vi "ConfigureWfrm.vi"(8 "error in (no error)":errorcluster, 10 "SampleRate":dbl=1000.0, 11 "PmuTestFunctions in":refnum<class "PmuTestFunctions.lvclass">) -> (0 "error out":errorcluster, 3 "PmuTestFunctions out":refnum<class "PmuTestFunctions.lvclass">)   [LabVIEW 2014, in "Functions.lvlib" / "PmuTestFunctions.lvclass"]
uses:
  PmuTestFunctions.lvclass
  ArbitraryFunction/ArbitraryFunction.lvclass/ArbitraryFunction.ctl
  PmuTestFunctions.lvclass/PmuTestFunctions.ctl
  ArbitraryFunction/Accessors/Read SampleRate.vi
  Accessors/Read PmuTestParams.vi
  Accessors/Read T0.vi
  ArbitraryFunction/Accessors/Read Arbs.vi
  Accessors/Read SettlingTime.vi
  ArbitraryFunction/Accessors/Write Arbs.vi
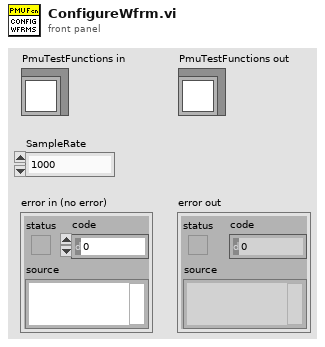
[diagram p1: front panel]
types:
  T1 = typedef "Functions.lvlib/PmuTestFunctions.lvclass/PmuTestParams.ctl" = dbl[][]
  T2 = typedef "Functions.lvlib/ArbitraryFunction.lvclass/Arbitrary.ctl" = cluster{"Handle":string, "Size":i32, "Gain":dbl, "Offset":dbl, "Waveform":waveform(dbl)}
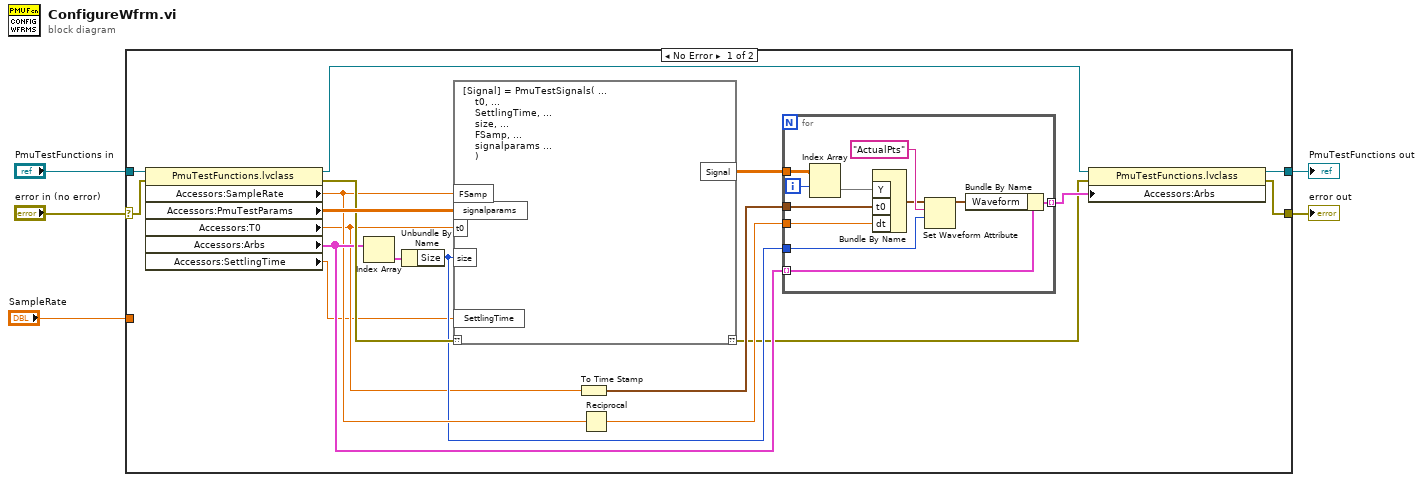
[diagram p0: block diagram]
diagram:
  n1 = case shown="No Error" "error in (no error)" {
    selector: "error in (no error)" -> [w22 w36]
    tunnel: [w7 w36] -> w4
    tunnel: [w8 w35] -> w2
    tunnel: "PmuTestFunctions in" -> [w23 w35]
    tunnel: "SampleRate" -> [_ _]
    frame No Error {
      n2 = property class="PmuTestFunctions.lvclass"(reference=w23, error in=w22) -> (reference out=w11:refnum<class "PmuTestFunctions.lvclass">, error out=w19:errorcluster, "Accessors:SampleRate"=w16:dbl, "Accessors:PmuTestParams"=w20:T1, "Accessors:T0"=w13:dbl, "Accessors:Arbs"=w18:T2[], "Accessors:SettlingTime"=w6:dbl)
      n3 = Index Array(array=w18) -> (element=w21:T2)  [unwired: 1 in]
      n4 = Unbundle By Name(w21) -> ("Size"=w14:i32)
      n5 = script code="[Signal] = PmuTestSignals( ...\n    t0, ...\n    SettlingTime, ...\n    size, ...\n    FSamp, ...\n    signalparams ...\n    )"("??"=w19, "t0"=w13, "size"=w14, "SettlingTime"=w6, "signalparams"=w20, "FSamp"=w16) -> ("??"=w9:errorcluster, "Signal"=w17:dbl[][])
      n6 = To Time Stamp(1:w13) -> (0:w12:timestamp)
      n7 = Reciprocal(x=w16) -> (1/x=w15:dbl)
      n8 = for {
        tunnel: w18 -> [w32] mode=indexing
        tunnel: w17 -> [w34]
        tunnel: w15 -> [w30]
        tunnel: w14 -> [w26]
        tunnel: w12 -> [w25]
        tunnel: [w24] -> w10 mode=indexing
        i -> [w33]
        n9 = Index Array(array=w34, index (row)=w33) -> (element=w31:dbl[])  [unwired: 1 in]
        n10 = Bundle By Name("Y"=w31, "t0"=w25, "dt"=w30) -> (w28:waveform(dbl))  [unwired: 1 in]
        n11 = Set Waveform Attribute(5:w26, 6:"ActualPts" ("name"), 7:w28) -> (3:w27:waveform(dbl))  [unwired: 1 in, 2 out]
        n12 = Bundle By Name(cluster=w32, "Waveform"=w27) -> (w24:T2)
      }
      n13 = property class="PmuTestFunctions.lvclass"(reference=w11, error in=w9, "Accessors:Arbs"=w10) -> (reference out=w8:refnum<class "PmuTestFunctions.lvclass">, error out=w7:errorcluster)
    }
    frame Error {
    }
  }
  "error out" <- w4
  "PmuTestFunctions out" <- w2
